vi "GFITS_FindImageFmList.vi"(8 "error in (no error)":errorcluster, 10 "Image":string, 11 "Path":path) -> (0 "error out":errorcluster, 2 "status":string)   [LabVIEW 2016]
uses:
  <vilib>/Utility/config.llb/Read Key (String).vi
  <vilib>/Utility/config.llb/NI_LVConfig.lvlib
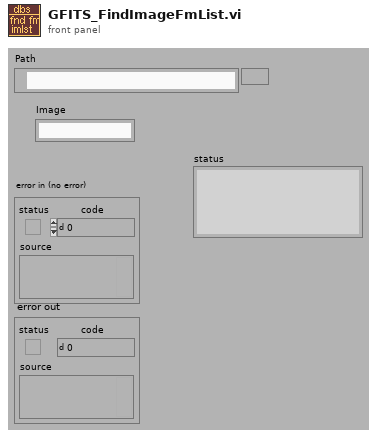
[diagram p1: front panel]
types:
  T1 = typedef "NI_LVConfig.lvlib/Config Data RefNum.ctl" = refnum<k1>
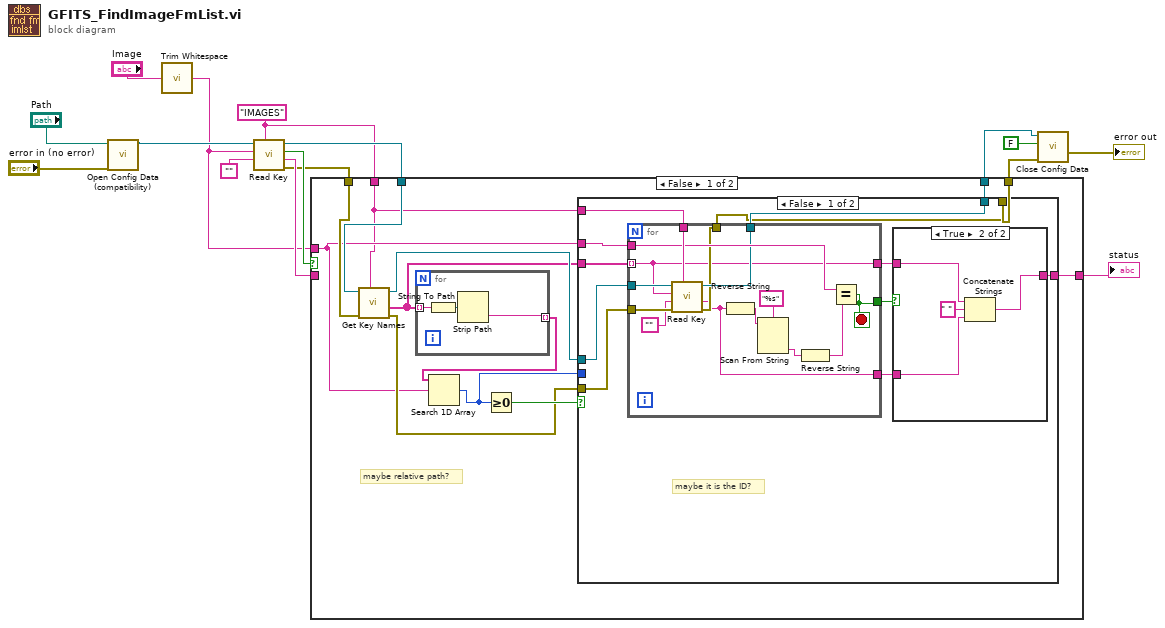
[diagram p0: block diagram]
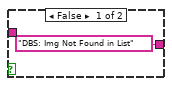
[diagram p2: hidden frame]
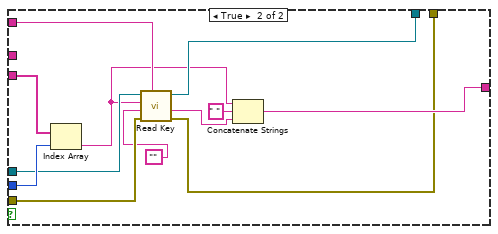
[diagram p3: hidden frame]
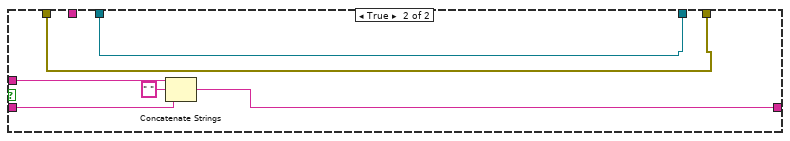
[diagram p4: hidden frame]
diagram:
  w1 = "IMAGES" ("section")
  n1 = call <vilib>:"Open Config Data (compatibility).vi"("error in (no error)"="error in (no error)", "configuration file path"="Path") -> ("refnum"=w13:T1)  [unwired: 7 in, 2 out]
  n2 = call <vilib>:"Trim Whitespace.vi"("string"="Image") -> ("trimmed string"=w7:string)  [unwired: 1 in]
  n3 = call-poly <vilib>:"Read Key.vi"("section"=w1, "default value"="", "key"=w7, "refnum"=w13) -> ("error out"=w4:errorcluster, "value"=w10:string, "found?"=w11:bool, "refnum out"=w5:T1)  [unwired: 2 in, 2 out]
  n4 = case shown="False" w11 {
    tunnel: w10 -> [_ w80]
    tunnel: [w29 w77] -> w9
    tunnel: w7 -> [w19 w78]
    tunnel: w5 -> [w26 w76]
    tunnel: w4 -> [w25 w75]
    tunnel: [w28 w75] -> w3
    tunnel: [w27 w76] -> w2
    tunnel: w1 -> [w17 _]
    frame False {
      # "maybe relative path?"
      n5 = call <vilib>:"Get Key Names.vi"("section"=w17, "error in (no error)"=w25, "refnum"=w26) -> ("error out"=w22:errorcluster, "key names"=w18:string[], "refnum out"=w23:T1)  [unwired: 6 out]
      n6 = for {
        tunnel: w18 -> [w31] mode=indexing
        tunnel: [w30] -> w21 mode=indexing
        n7 = String To Path(string=w31) -> (path=w32:path)
        n8 = Strip Path(path=w32) -> (name=w30:string)  [unwired: 1 out]
      }
      n9 = Search 1D Array(1D array=w21, element=w19) -> (index of element=w20:i32)  [unwired: 1 out]
      n10 = Greater Or Equal To 0?(x=w20) -> (x >= 0?=w24:bool)
      n11 = case shown="False" w24 {
        tunnel: [w43 w71] -> w29
        tunnel: w22 -> [w39 w68]
        tunnel: [w35 w66] -> w28
        tunnel: [w36 w67] -> w27
        tunnel: w23 -> [w40 w69]
        tunnel: w20 -> [_ w73]
        tunnel: w19 -> [w38 _]
        tunnel: w18 -> [w42 w72]
        tunnel: w17 -> [w41 w70]
        frame False {
          # "maybe it is the ID?"
          n12 = for {
            tunnel: w42 -> [w50] mode=indexing
            tunnel: w41 -> [w62]
            tunnel: w40 -> [w61]
            tunnel: w39 -> [w60]
            tunnel: w38 -> [w55]
            tunnel: [w53] -> w37
            tunnel: [w52] -> w36
            tunnel: [w51] -> w35
            tunnel: [w50] -> w34
            tunnel: [w49] -> w33
            stop <- w53 stop-if-true
            n13 = call-poly <vilib>:"Read Key.vi"("section"=w62, "error in (no error)"=w60, "default value"="", "key"=w50, "refnum"=w61) -> ("error out"=w51:errorcluster, "value"=w49:string, "refnum out"=w52:T1)  [unwired: 1 in, 3 out]
            n14 = Reverse String(1:w49) -> (0:w58:string)
            n15 = Scan From String(format string="%s", input string=w58) -> (output 1=w56:string)  [unwired: 2 in, 4 out]
            n16 = Reverse String(1:w56) -> (0:w54:string)
            n17 = Equal?(x=w55, y=w54) -> (x = y?=w53:bool)
          }
          n18 = case shown="True" w37 {
            tunnel: ["DBS: Img Not Found in List" w45] -> w43
            tunnel: w34 -> [_ w47]
            tunnel: w33 -> [_ w46]
            frame False {
            }
            frame True {
              n19 = Concatenate Strings(w47, " " ("string"), w46) -> (w45:string)
            }
          }
        }
        frame True {
          n20 = Index Array(array=w72, index=w73) -> (element=w65:string)
          n21 = call-poly <vilib>:"Read Key.vi"("section"=w70, "error in (no error)"=w68, "default value"="", "key"=w65, "refnum"=w69) -> ("error out"=w66:errorcluster, "value"=w63:string, "refnum out"=w67:T1)  [unwired: 1 in, 3 out]
          n22 = Concatenate Strings(w65, " " ("string"), w63) -> (w71:string)
        }
      }
    }
    frame True {
      n23 = Concatenate Strings(w78, " " ("string"), w80) -> (w77:string)
    }
  }
  "status" <- w9
  n24 = call <vilib>:"Close Config Data.vi"("error in (no error)"=w3, "write file if changed (T)"=FALSE ("write configuration file? (T)"), "refnum"=w2) -> ("error out"=→"error out":errorcluster)  [unwired: 8 out]
